vi "Close.vi"(8 "error in (no error)":errorcluster, 11 "SV_Publisher in":refnum<class "SV_Publisher.lvclass">) -> (0 "error out":errorcluster, 3 "SV_Publisher out":refnum<class "SV_Publisher.lvclass">)   [LabVIEW 2019, in "SV_Publisher.lvclass"]
uses:
  SV_Publisher.lvclass
  SV_Publisher.lvclass/SV_Publisher.ctl
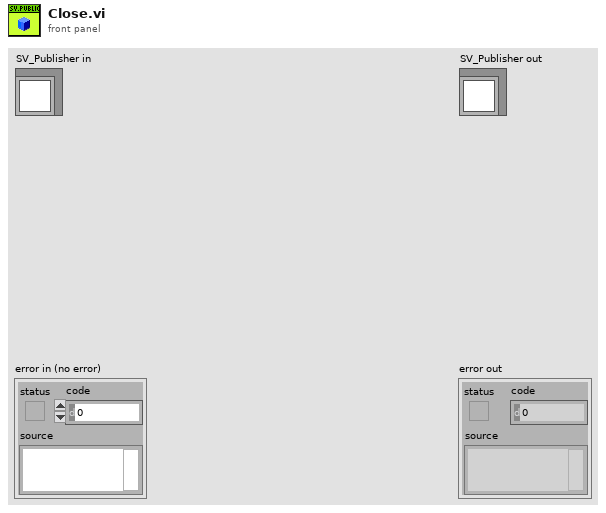
[diagram p1: front panel]
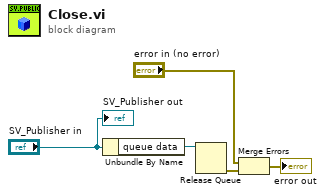
[diagram p0: block diagram]
diagram:
  n1 = Unbundle By Name("SV_Publisher in") -> ("queue data"=w3:refnum<queue>)
  n2 = Release Queue(queue=w3) -> (error out=w1:errorcluster)  [unwired: 2 in, 2 out]
  n3 = Merge Errors("error in (no error)", w1) -> (→"error out":errorcluster)
  "SV_Publisher out" <- "SV_Publisher in"
